vi "Semaphore.vi"() -> ()   [LabVIEW 2021]
uses:
  80be2e00-c6a9-3fb1-fe34-0b146306e83f.vi
  a82b5029-3aca-3fcb-08ce-400ad2ebd73f.vi
panel:
  in  "Numeric":i32
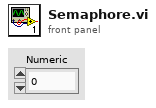
[diagram p1: front panel]
types:
  T1 = typedef "Semaphore RefNum" = refnum<k1>
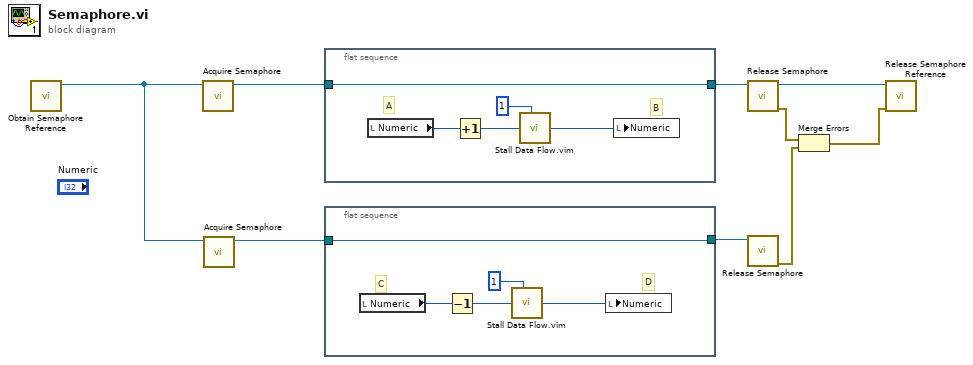
[diagram p0: block diagram]
diagram:
  n1 = call <vilib>:"Obtain Semaphore Reference.vi"() -> ("semaphore"=w7:T1)  [unwired: 5 in, 2 out]
  n2 = call <vilib>:"Acquire Semaphore.vi"("semaphore"=w7) -> ("semaphore out"=w9:T1)  [unwired: 4 in, 2 out]
  n3 = call <vilib>:"Acquire Semaphore.vi"("semaphore"=w7) -> ("semaphore out"=w6:T1)  [unwired: 4 in, 2 out]
  n4 = flat-sequence {
    tunnel: w9 -> [w10]
    tunnel: [w10] -> w8
    frame #0 {
      # "B"
      # "A"
      n5 = local read "Numeric"() -> (w11:i32)
      n6 = Increment(x=w11) -> (x+1=w12:i32)
      n7 = call "Stall Data Flow.vim"("value in"=w12, "milliseconds to wait"=u32 1) -> ("value out"=w13:i32)  [unwired: 1 out]
      n8 = local write "Numeric"(w13) -> ()
    }
  }
  n9 = flat-sequence {
    tunnel: [w15] -> w5
    tunnel: w6 -> [w15]
    frame #0 {
      # "D"
      # "C"
      n10 = local read "Numeric"() -> (w16:i32)
      n11 = Decrement(x=w16) -> (x-1=w17:i32)
      n12 = call "Stall Data Flow.vim"("value in"=w17, "milliseconds to wait"=u32 1) -> ("value out"=w18:i32)  [unwired: 1 out]
      n13 = local write "Numeric"(w18) -> ()
    }
  }
  n14 = call <vilib>:"Release Semaphore.vi"("semaphore"=w8) -> ("error out"=w4:errorcluster, "semaphore out"=w2:T1)  [unwired: 5 in]
  n15 = call <vilib>:"Release Semaphore.vi"("semaphore"=w5) -> ("error out"=w3:errorcluster)  [unwired: 5 in, 1 out]
  n16 = Merge Errors "Merge Errors"(w4, w3) -> (w1:errorcluster)
  n17 = call <vilib>:"Release Semaphore Reference.vi"("error in (no error)"=w1, "semaphore"=w2) -> ()  [unwired: 8 in, 2 out]
